vi "ConfigGUID to ChannelNodeID.vi"(8 "error in":errorcluster, 10 "ConfigGUID Linkages":T2[](array[typedef]), 11 "Response in":T1 format="%.0x") -> (0 "error out":errorcluster, 2 "NodeID Linkages":T3[](array[typedef]) {"Channel Refnum" format="%.0x"}, 3 "Response out":T1=18446744073709551615 format="%.0x")   [LabVIEW 2018, in "Instrument Addon Scripting API.lvlib"]
uses:
  Instrument Addon Scripting API.lvlib
  <vilib>/NI Veristand/Custom Device API/Custom Device Item Ref.ctl
  TypeDefs/Linked Channel.ctl
  Addon/Addon Shared/Types/Linked Channel Cluster.ctl
  Addon/Addon Shared/SubVIs/Constants.vi
  <vilib>/NI Veristand/Custom Device API/Get Item Property (String).vi
  <vilib>/NI Veristand/Custom Device API/Custom Device API.lvlib
  Addon/Addon Shared/Instrument Addon Shared.lvlib
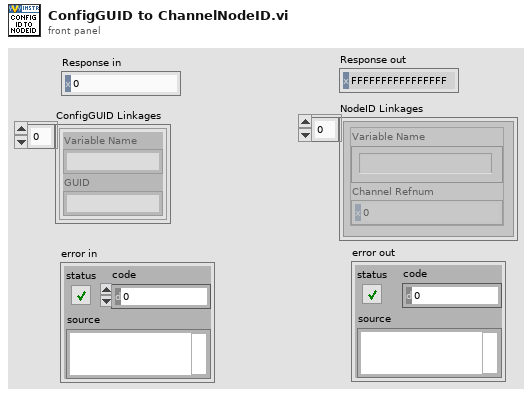
[diagram p1: front panel]
types:
  T1 = typedef "Custom Device API.lvlib/Custom Device Item Ref.ctl" = u64
  T2 = typedef "Instrument Addon Shared.lvlib/Linked Channel Cluster.ctl" = cluster{"Variable Name":string, "GUID":string}
  T3 = typedef "Instrument Addon Scripting API.lvlib/Linked Channel.ctl" = cluster{"Variable Name":string, "Channel Refnum":T1}
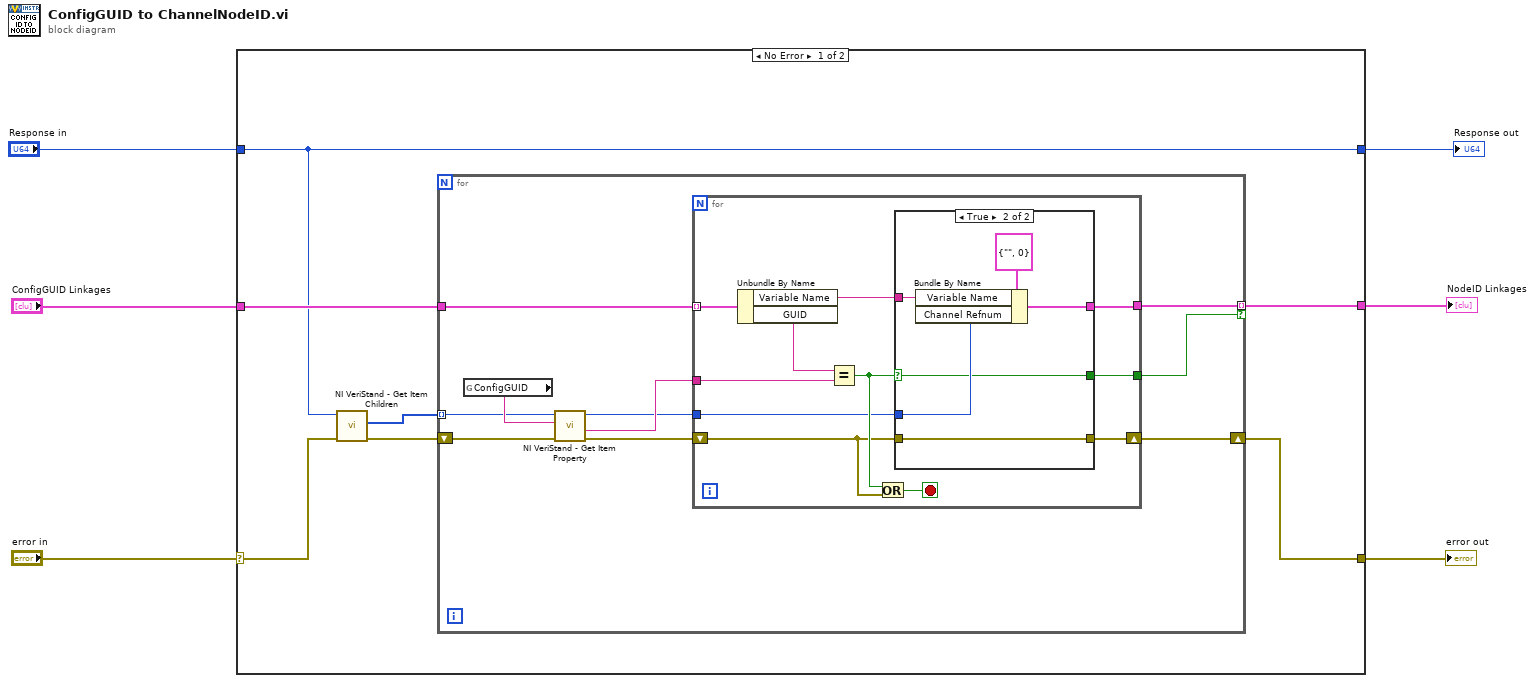
[diagram p0: block diagram]
diagram:
  n1 = case shown="No Error" "error in" {
    selector: "error in" -> [w8 w44]
    tunnel: "Response in" -> [w7 w43]
    tunnel: "ConfigGUID Linkages" -> [w11 _]
    tunnel: [w10 w44] -> w4
    tunnel: [w9 _] -> w3
    tunnel: [w7 w43] -> w1
    frame No Error {
      n2 = call <vilib>:"NI VeriStand - Get Item Children.vi"("error in (no error)"=w8, "Item Ref in"=w7) -> ("error out"=w12:errorcluster, "Child Refs"=w13:T1[])  [unwired: 6 in, 2 out]
      n3 = for {
        tunnel: w13 -> [w21] mode=indexing
        shift-right: [w14] -> w10
        shift-left: w12 -> [w22]
        tunnel: w11 -> [w18]
        tunnel: [w16] -> w9 mode=indexing if=w15
        n4 = global read "Constants.vi" "ConfigGUID"() -> (w23:string)
        n5 = call-poly <vilib>:"NI VeriStand - Get Item Property.vi"("error in (no error)"=w22, "Property Name"=w23, "Item Ref in"=w21) -> ("error out"=w19:errorcluster, "Value"=w20:string, "Item Ref out"=w17:T1)  [unwired: 5 in, 1 out]
        n6 = for {
          tunnel: w20 -> [w34]
          tunnel: w18 -> [w33] mode=indexing
          tunnel: w17 -> [w29]
          shift-right: [w24] -> w14
          shift-left: w19 -> [w25]
          tunnel: [w27] -> w16
          tunnel: [w26] -> w15
          stop <- w31 stop-if-true
          n7 = Unbundle By Name(w33) -> ("Variable Name"=w28:string, "GUID"=w32:string)
          n8 = Equal?(x=w32, y=w34) -> (x = y?=w30:bool)
          n9 = Or(x=w30, y=w25) -> (x .or. y?=w31:bool)
          n10 = case shown="True" w30 {
            selector: w30 -> [w36 w38]
            tunnel: w29 -> [_ w40]
            tunnel: w28 -> [_ w41]
            tunnel: [_ w39] -> w27
            tunnel: [w36 w38] -> w26
            tunnel: w25 -> [w35 w37]
            tunnel: [w35 w37] -> w24
            frame False {
            }
            frame True {
              n11 = Bundle By Name(cluster=T3 {"Variable Name"="", "Channel Refnum"=0} ("Linked Channel"), "Variable Name"=w41, "Channel Refnum"=w40) -> (w39:T3)
            }
          }
        }
      }
    }
    frame Error {
    }
  }
  "error out" <- w4
  "NodeID Linkages" <- w3
  "Response out" <- w1
